vi "Data Types Base Directory.vi"(8 "error in":errorcluster, 10 "Data Types Directory":path) -> (0 "error out":errorcluster)   [LabVIEW 2020, in "Data Type Scripting.lvlib"]
doc: "_____\nCreated using DQMH Event Scripter 6.0.0.122."
uses:
  Data Type Scripting.lvlib
  Data Types Base Directory Argument--cluster.ctl
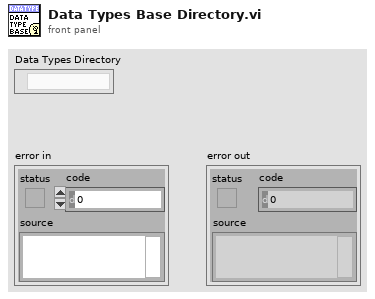
[diagram p1: front panel]
types:
  T1 = typedef "Data Type Scripting.lvlib/Data Types Base Directory Argument--cluster.ctl" = cluster{"Data Types Directory":path}
  T2 = typedef "Data Type Scripting.lvlib/Broadcast Events--cluster.ctl" = cluster{"Module Did Init":refnum<user-event>, "Status Updated":refnum<user-event>, "Error Reported":refnum<user-event>, "Module Did Stop":refnum<user-event>, "Update Module Execution Status":refnum<user-event>, "Template Path":refnum<user-event>, "Poly List":refnum<user-event>, "Poly Details":refnum<user-event>, "Data Type Valid":refnum<user-event>, "List of Data Types":refnum<user-event>, "Data Type Created":refnum<user-event>, "Selected Edit Data Type Info":refnum<user-event>, "Data Types Base Directory":refnum<user-event>}
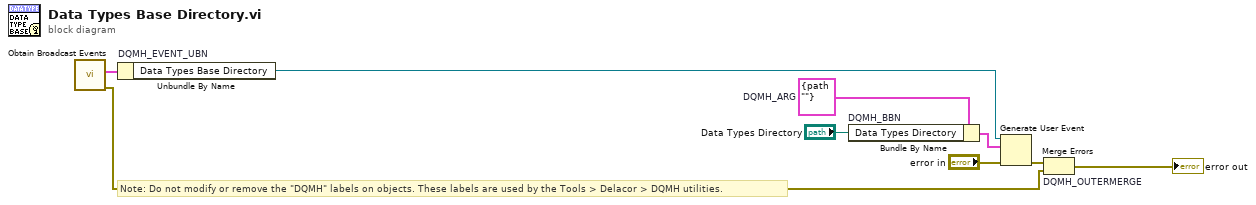
[diagram p0: block diagram]
diagram:
  w4 = T1 {"Data Types Directory"=path ""}  # DQMH_ARG
  # "Note: Do not modify or remove the \"DQMH\" labels on objects. These labels are used by the Tools > Delacor > DQMH utilities."
  n1 = call "Obtain Broadcast Events.vi"() -> ("error out"=w2:errorcluster, "Data Type Scripting Broadcast Events"=w1:T2)  [unwired: 10 in]
  n2 = Unbundle By Name "DQMH_EVENT_UBN"(w1) -> ("Data Types Base Directory"=w6:refnum<user-event>)
  n3 = Bundle By Name "DQMH_BBN"(cluster=w4, "Data Types Directory"="Data Types Directory") -> (w7:T1)
  n4 = Generate User Event(user event=w6, event data cluster=w7, error in="error in") -> (error out=w5:errorcluster)  [unwired: 1 in, 1 out]
  n5 = Merge Errors "DQMH_OUTERMERGE"(w5, w2) -> (→"error out":errorcluster)
